vi "IFD Additional Info.vi"(8 "error in (no error)":errorcluster, 9 "Page":cluster{"Total Pages":u16, "Current Page":u16}, 10 "Is ref?":bool, 11 "IFD in":refnum<class "IFD.lvclass">) -> (0 "error out":errorcluster, 3 "IFD out":refnum<class "IFD.lvclass">)   [LabVIEW 2016, in "IFD.lvclass"]
uses:
  IFD.lvclass
  Tag/IFD_Tag.lvclass/IFD_Tag.ctl
  Tag/IFD_Tag.lvclass
  IFD.lvclass/IFD.ctl
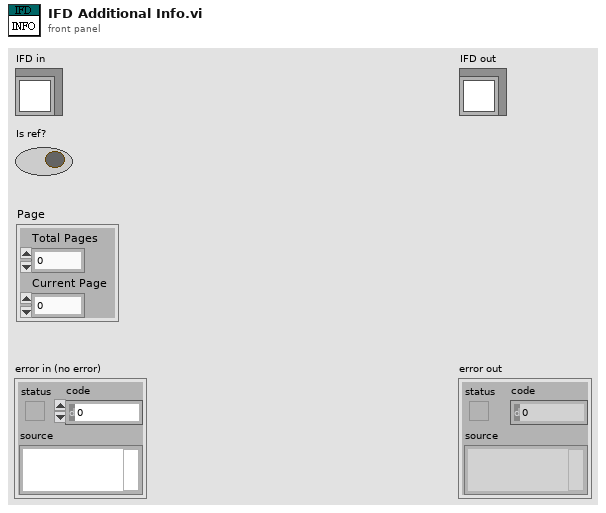
[diagram p1: front panel]
types:
  T1 = enum16{"Undefined(DO NOT USE)", "U8", "ASCII", "U16", "U32", "RATIONAL", "I8", "Undefined 8 bit", "I16", "I32", "SRATIONAL", "SGL", "DBL"}
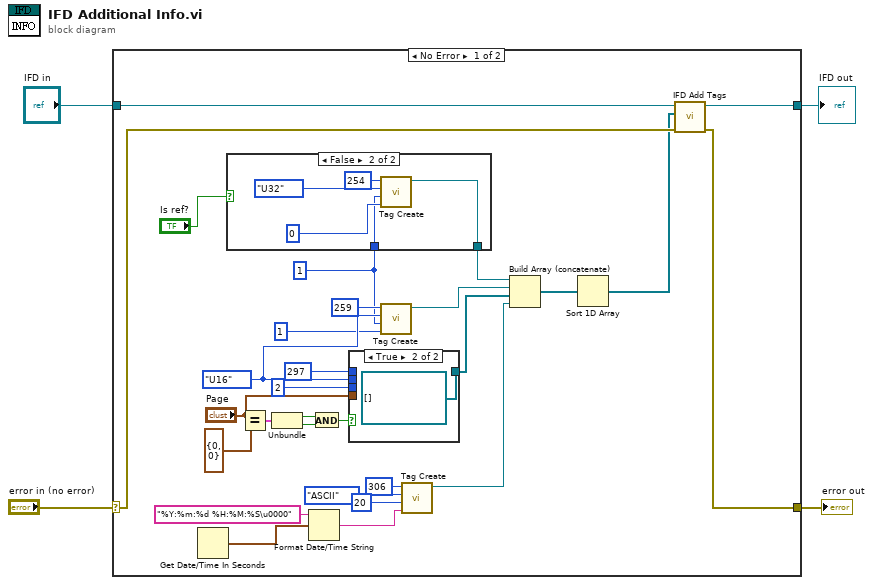
[diagram p0: block diagram]
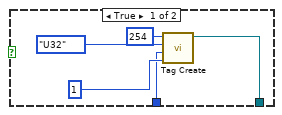
[diagram p2: hidden frame]
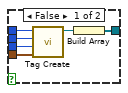
[diagram p3: hidden frame]
diagram:
  n1 = case shown="No Error" "error in (no error)" {
    selector: "error in (no error)" -> [w25 w52]
    tunnel: [w24 w52] -> w3
    tunnel: [w32 w51] -> w1
    tunnel: "IFD in" -> [w33 w51]
    frame No Error {
      w7 = u32 1 ("Data Count")
      w20 = T1."U16" ("Data Type")
      n2 = Get Date/Time In Seconds() -> (seconds since 1Jan1904=w30:timestamp)
      n3 = case shown="False" "Is ref?" {
        tunnel: w7 -> [w35 w40]
        tunnel: [w34 w39] -> w18
        frame True {
          n4 = call "Tag Create.vi"("Data"=u32 1, "Data Count"=w35, "Data Type"=T1."U32", "Tag ID"=u16 254) -> ("IFD_Tag out"=w34:refnum<class "IFD_Tag.lvclass">)  [unwired: 7 in]
        }
        frame False {
          n5 = call "Tag Create.vi"("Data"=u32 0, "Data Count"=w40, "Data Type"=T1."U32", "Tag ID"=u16 254) -> ("IFD_Tag out"=w39:refnum<class "IFD_Tag.lvclass">)  [unwired: 7 in]
        }
      }
      n6 = Equal?(x="Page", y=cluster{"Total Pages":u16, "Current Page":u16} {"Total Pages"=0, "Current Page"=0}) -> (x = y?=w11:cluster{"Total Pages":bool, "Current Page":bool})
      n7 = Unbundle(w11) -> ("Total Pages"=w10:bool, "Current Page"=w9:bool)
      n8 = Format Date/Time String(time format string (%c)="%Y:%m:%d %H:%M:%S\u0000", seconds (now)=w30) -> (date/time string=w26:string)  [unwired: 1 in]
      n9 = And(x=w10, y=w9) -> (x .and. y?=w8:bool)
      n10 = case shown="True" w8 {
        tunnel: u16 297 ("Tag ID") -> [w49 _]
        tunnel: u32 2 ("Data Count") -> [w48 _]
        tunnel: w20 -> [w47 _]
        tunnel: [w44 refnum<class "IFD_Tag.lvclass">[] []] -> w16
        tunnel: "Page" -> [w46 _]
        frame False {
          n11 = call "Tag Create.vi"("Data"=w46, "Data Count"=w48, "Data Type"=w47, "Tag ID"=w49) -> ("IFD_Tag out"=w45:refnum<class "IFD_Tag.lvclass">)  [unwired: 7 in]
          n12 = Build Array(w45) -> (w44:refnum<class "IFD_Tag.lvclass">[])
        }
        frame True {
        }
      }
      n13 = call "Tag Create.vi"("Data"=u16 1, "Data Count"=w7, "Data Type"=w20, "Tag ID"=u16 259) -> ("IFD_Tag out"=w17:refnum<class "IFD_Tag.lvclass">)  [unwired: 7 in]
      n14 = call "Tag Create.vi"("Data"=w26, "Data Count"=u32 20, "Data Type"=T1."ASCII", "Tag ID"=u16 306) -> ("IFD_Tag out"=w15:refnum<class "IFD_Tag.lvclass">)  [unwired: 7 in]
      n15 = Build Array (concatenate)(w18, w17, w16, w15) -> (w14:refnum<class "IFD_Tag.lvclass">[])
      n16 = Sort 1D Array(array=w14) -> (sorted array=w5:refnum<class "IFD_Tag.lvclass">[])
      n17 = call "IFD Add Tags.vi"("error in (no error)"=w25, "Tag(s)"=w5, "IFD in"=w33) -> ("error out"=w24:errorcluster, "IFD out"=w32:refnum<class "IFD.lvclass">)  [unwired: 7 in]
    }
    frame Error {
    }
  }
  "error out" <- w3
  "IFD out" <- w1
